vi "Main-Centering DNA Tether_YCC.vi"() -> ()   [LabVIEW 2014]
uses:
  Main-Stage-PI/(Global) Current handle and LaserPower_YCC.vi
  <vilib>/DAQmx/configure/timing.llb/DAQmx Timing (Sample Clock).vi
  <vilib>/DAQmx/create/channels.llb/DAQmx Create Channel (AI-Voltage-Basic).vi
  <vilib>/DAQmx/read.llb/DAQmx Read (Analog 2D DBL NChan NSamp).vi
  <vilib>/Utility/file.llb/Write To Spreadsheet File (DBL).vi
panel:
  out "Filtered QPD data":dbl[](array[numeric])
  out "Filtered Stage Array":dbl[](array[numeric])
  in  "Save Data?":bool
  out "Running time":dbl
  in  "Move to new Center?":bool
  in  "no record \nscan rate  (um/s)":dbl=4.0
  out "need time":dbl
  out "True rate?":bool
  out "x*y 2":dbl
  out "x-y":dbl
  out "Sample points want to record":dbl
  out "Center":dbl
  out "min":dbl
  out "Max":dbl
  out "Numeric":dbl
  out "Move to":dbl
  in  "Tab Control":enum32{"Filter", "Raw+Filter"}(tab)
  out "Filtered stage-QPD Graph":cluster{dbl[], "Filtered X":dbl[]}(graph)
  out "Raw+Filter stage-QPD Graph":cluster{"Raw Stage Array":dbl[], "data":dbl[]}[](graph)
  in  "Filter type":T1(ring)
  in  "Avg points":i32
  out "Stage Array from one end to the other end":dbl[](array[numeric])
  out "total time to travel (s)":dbl
  out "Axis":i32
  in  "T=+ first\nF=- first":bool
  out "Real initial position (um)":dbl format="%0.5f"
  in  "Maximum Value":dbl=1.0 format="%0.2f"
  in  "Minimum Value":dbl=-1.0 format="%0.2f"
  in  "Sampling rate (Hz)":dbl=20000.0 format="%0.2f"
  in  "scan rate  (um/s)":dbl=2.0 format="%.3f"
  in  "Scan Range  (um)":dbl=2.0 format="%.3f"
  in  "X=T,Y=F":bool
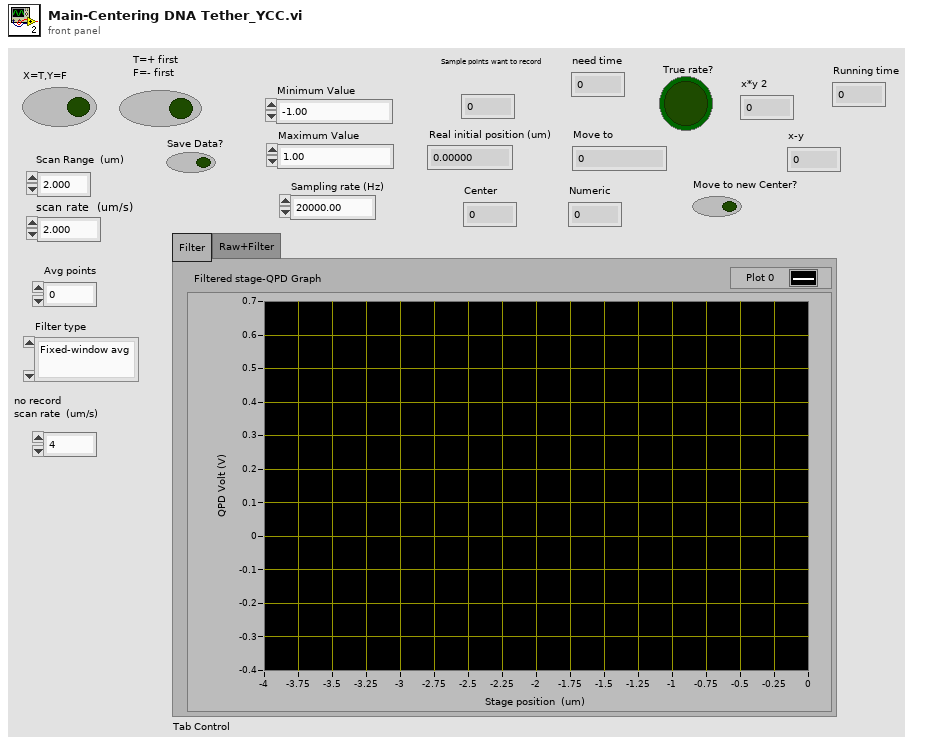
[diagram p1: front panel]
types:
  T1 = enum16{"Fixed-window avg", "Moving-window avg", "S-G filter", "Median filter"}
  T2 = cluster{"Filtered Stage Array":dbl[], "Filtered QPD data":dbl[]}
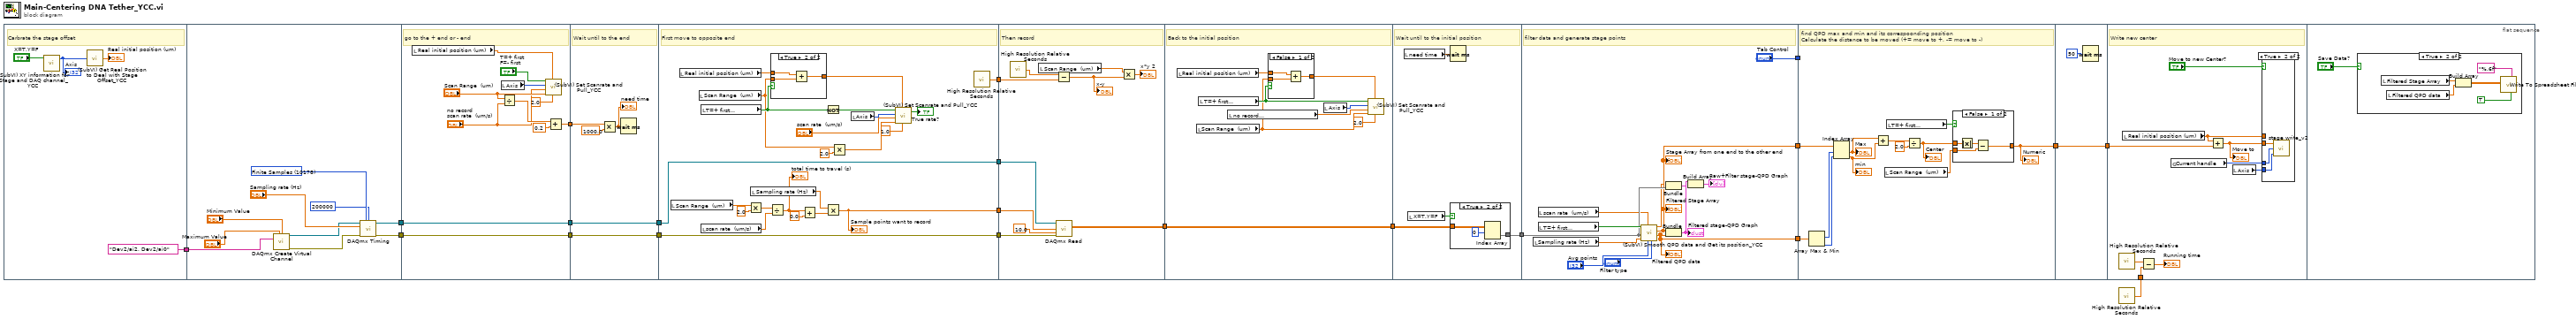
[diagram p0: block diagram]
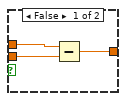
[diagram p2: hidden frame]
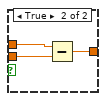
[diagram p3: hidden frame]
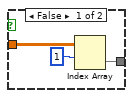
[diagram p4: hidden frame]
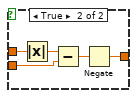
[diagram p5: hidden frame]
diagram:
  n1 = flat-sequence {
    tunnel: [tag "Dev2/ai2, Dev2/ai0" ("physical channels")] -> w21
    tunnel: w21 -> [w29]
    tunnel: [w28] -> w13
    tunnel: [w27] -> w11
    tunnel: [w41] -> w15
    tunnel: [w40] -> w14
    tunnel: w13 -> [w40]
    tunnel: [w39] -> w12
    tunnel: w11 -> [w39]
    tunnel: w15 -> [w51]
    tunnel: [w48] -> w3
    tunnel: w14 -> [w48]
    tunnel: [w47] -> w2
    tunnel: w12 -> [w47]
    tunnel: [w57] -> w7
    tunnel: w3 -> [w74]
    tunnel: [w74] -> w6
    tunnel: w2 -> [w73]
    tunnel: [w73] -> w5
    tunnel: [w72] -> w4
    tunnel: [w90] -> w10
    tunnel: w7 -> [w89]
    tunnel: w6 -> [w83]
    tunnel: w5 -> [w81]
    tunnel: w4 -> [w87]
    tunnel: w10 -> [w98]
    tunnel: [w98] -> w9
    tunnel: w9 -> [w107]
    tunnel: [w105] -> w8
    tunnel: w8 -> [w125]
    tunnel: [w119] -> w20
    tunnel: [w120] -> w19
    tunnel: ["Tab Control"] -> w18
    tunnel: w20 -> [w139]
    tunnel: w19 -> [w138]
    tunnel: [w128] -> w17
    tunnel: w18 -> [_]
    tunnel: w17 -> [w150]
    tunnel: [w150] -> w16
    tunnel: w16 -> [w154]
    tunnel: w1 -> [w152]
    frame #0 {
      # "Carbrate the stage offset"
      n2 = call "(SubVI) XY information for Stage and DAQ channel_YCC.vi"("T=X\nF=Y"="X=T,Y=F") -> ("Axis"=w23:i32)  [unwired: 3 in, 1 out]
      "Axis" <- w23
      n3 = call "(SubVI) Get Real Position to Deal with Stage Offset_YCC.vi"("Axis"=w23) -> ("Real Current Commanded position (um)"=→"Real initial position (um)":dbl)  [unwired: 3 in, 1 out]
    }
    frame #1 {
      w33 = 10178 items=["Finite Samples"=10178, "Continuous Samples"=10123, "Hardware Timed Single Point"=12522] ("sample mode")
      n4 = call-poly <vilib>:"DAQmx Create Virtual Channel.vi"("maximum value"="Maximum Value", "minimum value"="Minimum Value", "physical channels"=w29) -> ("task out"=w32:refnum<k21>, "error out"=w35:errorcluster)  [unwired: 6 in, 5 out]
      n5 = call-poly <vilib>:"DAQmx Timing.vi"("task/channels in"=w32, "sample mode"=w33, "samples per channel"=200000, "rate"="Sampling rate (Hz)", "error in"=w35) -> ("task out"=w28:refnum<k21>, "error out"=w27:errorcluster)  [unwired: 9 in]
    }
    frame #2 {
      # "go to the + end or - end"
      n6 = local read "Real initial position (um)"() -> (w37:dbl)
      n7 = local read "Axis"() -> (w46:i32)
      n8 = Divide(x="Scan Range  (um)", y="no record \nscan rate  (um/s)") -> (x/y=w43:dbl)
      n9 = call "(SubVI) Set Scanrate and Pull_YCC.vi"("waiting time per point (ms)\nrange from 5ms to 0.167 ms"=2.0 ("waiting time per point (ms)\nrange from 5ms to 0.167 ms"), "Start From  (um)"=w37, "range  (um)"="Scan Range  (um)", "scan rate  (um/s)"="no record \nscan rate  (um/s)", "axis"=w46, "toward+ ?\nT=+, F=-"="T=+ first\nF=- first") -> ()  [unwired: 2 out]
      n10 = Add(x=w43, y=0.2) -> (x+y=w41:dbl)
    }
    frame #3 {
      # "Wait until to the end"
      n11 = Multiply(x=w51, y=1000.0) -> (x*y=w49:dbl)
      "need time" <- w49
      n12 = Wait (ms)(milliseconds to wait=w49) -> ()  [unwired: 1 out]
    }
    frame #4 {
      # "First move to opposite end"
      n13 = local read "Scan Range  (um)"() -> (w59:dbl)
      n14 = local read "Real initial position (um)"() -> (w54:dbl)
      n15 = local read "Scan Range  (um)"() -> (w53:dbl)
      n16 = local read "T=+ first\nF=- first"() -> (w55:bool)
      n17 = local read "scan rate  (um/s)"() -> (w58:dbl)
      n18 = Multiply(x=w59, y=2.0) -> (x*y=w61:dbl)
      n19 = local read "Sampling rate (Hz)"() -> (w62:dbl)
      n20 = Divide(x=w61, y=w58) -> (x/y=w63:dbl)
      "total time to travel (s)" <- w63
      n21 = case shown="True" w55 {
        tunnel: w54 -> [w77 w80]
        tunnel: w53 -> [w76 w79]
        tunnel: [w75 w78] -> w52
        frame False {
          n22 = Subtract(x=w77, y=w76) -> (x-y=w75:dbl)
        }
        frame True {
          n23 = Add(x=w80, y=w79) -> (x+y=w78:dbl)
        }
      }
      n24 = Add(x=w63, y=0.0) -> (x+y=w64:dbl)
      n25 = Not(x=w55) -> (.not. x?=w66:bool)
      n26 = Multiply(x=w62, y=w64) -> (x*y=w57:dbl)
      "Sample points want to record" <- w57
      n27 = Multiply(x=w53, y=2.0) -> (x*y=w67:dbl)
      n28 = local read "Axis"() -> (w56:i32)
      n29 = call "(SubVI) Set Scanrate and Pull_YCC.vi"("waiting time per point (ms)\nrange from 5ms to 0.167 ms"=1.0 ("waiting time per point (ms)\nrange from 5ms to 0.167 ms"), "Start From  (um)"=w52, "range  (um)"=w67, "scan rate  (um/s)"="scan rate  (um/s)", "axis"=w56, "toward+ ?\nT=+, F=-"=w66) -> ("True rate?"=→"True rate?":bool)  [unwired: 1 out]
      n30 = call <vilib>:"High Resolution Relative Seconds.vi"() -> ("relative seconds"=w72:dbl)
    }
    frame #5 {
      # "Then record"
      n31 = call <vilib>:"High Resolution Relative Seconds.vi"() -> ("relative seconds"=w88:dbl)
      n32 = local read "Scan Range  (um)"() -> (w86:dbl)
      n33 = Subtract(x=w88, y=w87) -> (x-y=w85:dbl)
      "x-y" <- w85
      n34 = call-poly <vilib>:"DAQmx Read.vi"("task/channels in"=w83, "number of samples per channel"=w89, "timeout"=10.0, "error in"=w81) -> ("data"=w90:dbl[][])  [unwired: 9 in, 2 out]
      n35 = Multiply(x=w86, y=w85) -> (x*y=→"x*y 2":dbl)
    }
    frame #6 {
      # "Back to the initial position"
      n36 = local read "Real initial position (um)"() -> (w93:dbl)
      n37 = local read "Scan Range  (um)"() -> (w92:dbl)
      n38 = local read "T=+ first\nF=- first"() -> (w94:bool)
      n39 = local read "no record \nscan rate  (um/s)"() -> (w96:dbl)
      n40 = case shown="False" w94 {
        tunnel: [w101 w104] -> w91
        tunnel: w93 -> [w100 w103]
        tunnel: w92 -> [w99 w102]
        frame False {
          n41 = Add(x=w100, y=w99) -> (x+y=w101:dbl)
        }
        frame True {
          n42 = Subtract(x=w103, y=w102) -> (x-y=w104:dbl)
        }
      }
      n43 = local read "Axis"() -> (w95:i32)
      n44 = call "(SubVI) Set Scanrate and Pull_YCC.vi"("waiting time per point (ms)\nrange from 5ms to 0.167 ms"=2.0 ("waiting time per point (ms)\nrange from 5ms to 0.167 ms"), "Start From  (um)"=w91, "range  (um)"=w92, "scan rate  (um/s)"=w96, "axis"=w95, "toward+ ?\nT=+, F=-"=w94) -> ()  [unwired: 2 out]
    }
    frame #7 {
      # "Wait until to the initial position"
      n45 = local read "need time"() -> (w108:dbl)
      n46 = local read "X=T,Y=F"() -> (w106:bool)
      n47 = Wait (ms)(milliseconds to wait=w108) -> ()  [unwired: 1 out]
      n48 = case shown="True" w106 {
        tunnel: w107 -> [w110 w114]
        tunnel: [w109 w112] -> w105
        frame False {
          n49 = Index Array(array=w110, index (row)=1) -> (element=w109:dbl[])  [unwired: 1 in]
        }
        frame True {
          n50 = Index Array(array=w114, index (row)=0) -> (element=w112:dbl[])  [unwired: 1 in]
        }
      }
    }
    frame #8 {
      # "filter data and generate stage points"
      n51 = local read "Sampling rate (Hz)"() -> (w124:dbl)
      n52 = local read "scan rate  (um/s)"() -> (w123:dbl)
      n53 = local read "T=+ first\nF=- first"() -> (w126:bool)
      n54 = call "(SubVI) Smooth QPD data and Get its position_YCC.vi"("Filter type"="Filter type", "Avg points"="Avg points", "scan rate  (um/s)"=w123, "Sampling rate (Hz)"=w124, "QPD data"=w125, "Direction\nT=+ \nF=-"=w126) -> ("Filtered QPD data"=w119:dbl[], "Filtered Stage Array"=w120:dbl[], "Raw Stage Array"=w118:dbl[])  [unwired: 3 in]
      "Stage Array from one end to the other end" <- w120
      "Filtered Stage Array" <- w120
      "Filtered QPD data" <- w119
      n55 = Bundle("Raw Stage Array"=w118, "data"=w125) -> (w116:cluster{"Raw Stage Array":dbl[], "data":dbl[]})  [unwired: 1 in]
      n56 = Bundle("Filtered Stage Array"=w120, "Filtered QPD data"=w119) -> (w117:T2)  [unwired: 1 in]
      "Filtered stage-QPD Graph" <- w117
      n57 = Build Array(w117, w116) -> (→"Raw+Filter stage-QPD Graph":cluster{"Raw Stage Array":dbl[], "data":dbl[]}[])
    }
    frame #9 {
      # "find QPD max and min and its correspoonding position\nCalculate the distance to be moved (+= move to +, -= move to -)"
      n58 = Array Max & Min(array=w139) -> (max index (indices)=w135:i32, min index (indices)=w134:i32)  [unwired: 2 out]
      n59 = Index Array(array=w138, index #1=w135, index #2=w134) -> (element #1=w133:dbl, element #2=w132:dbl)
      "Max" <- w133
      "min" <- w132
      n60 = Add(x=w133, y=w132) -> (x+y=w137:dbl)
      n61 = local read "Scan Range  (um)"() -> (w130:dbl)
      n62 = local read "T=+ first\nF=- first"() -> (w131:bool)
      n63 = Divide(x=w137, y=2.0) -> (x/y=w129:dbl)
      "Center" <- w129
      n64 = case shown="False" w131 {
        tunnel: w130 -> [w143 w148]
        tunnel: w129 -> [w141 w145]
        tunnel: [w142 w147] -> w128
        frame False {
          n65 = Absolute Value(x=w141) -> (abs(x)=w140:dbl)
          n66 = Subtract(x=w140, y=w143) -> (x-y=w142:dbl)
        }
        frame True {
          n67 = Absolute Value(x=w145) -> (abs(x)=w144:dbl)
          n68 = Subtract(x=w144, y=w148) -> (x-y=w146:dbl)
          n69 = Negate(x=w146) -> (-x=w147:dbl)
        }
      }
      "Numeric" <- w128
    }
    frame #10 {
      n70 = Wait (ms)(milliseconds to wait=u32 50) -> ()  [unwired: 1 out]
    }
    frame #11 {
      # "Write new center"
      n71 = call <vilib>:"High Resolution Relative Seconds.vi"() -> ("relative seconds"=w153:dbl)
      n72 = local read "Real initial position (um)"() -> (w155:dbl)
      n73 = Subtract(x=w153, y=w152) -> (x-y=→"Running time":dbl)
      n74 = global read "(Global) Current handle and LaserPower_YCC.vi" "Current handle"() -> (w157:i32)
      n75 = Add(x=w155, y=w154) -> (x+y=w158:dbl)
      "Move to" <- w158
      n76 = local read "Axis"() -> (w156:i32)
      n77 = case shown="True" "Move to new Center?" {
        tunnel: w158 -> [_ w162]
        tunnel: w157 -> [_ w161]
        tunnel: w156 -> [_ w160]
        tunnel: w155 -> [_ _]
        frame False {
        }
        frame True {
          n78 = call "stage write_v2.vi"("axis"=w160, "Incoming Handle"=w161, "position"=w162) -> ()  [unwired: 2 in, 1 out]
        }
      }
    }
    frame #12 {
      n79 = case shown="True" "Save Data?" {
        frame False {
        }
        frame True {
          n80 = local read "Filtered Stage Array"() -> (w168:dbl[])
          n81 = local read "Filtered QPD data"() -> (w167:dbl[])
          n82 = Build Array(w168, w167) -> (w166:dbl[][])
          n83 = call-poly <vilib>:"Write To Spreadsheet File.vi"("transpose? (no:F)"=TRUE, "format (%.3f)"="%.6f", "2D data"=w166) -> ()  [unwired: 5 in, 1 out]
        }
      }
    }
  }
  n84 = call <vilib>:"High Resolution Relative Seconds.vi"() -> ("relative seconds"=w1:dbl)
